vi "correlation tester.vi"() -> ()   [LabVIEW 2012]
uses:
  <vilib>/Utility/file.llb/Write To Spreadsheet File (DBL).vi
  <vilib>/vision/NI_Vision_Development_Module.lvlib
panel:
  in  "cc?":bool
  in  "report file name":path
  in  "error in":errorcluster
  out "error out":errorcluster
  out "Alignement peak":i32[](graph)
  out "Maximum quality per image":dbl[](graph)
  out "Alignment quality profile":sgl[](graph)
  in  "background image":path
  in  "Image sequence folder":path
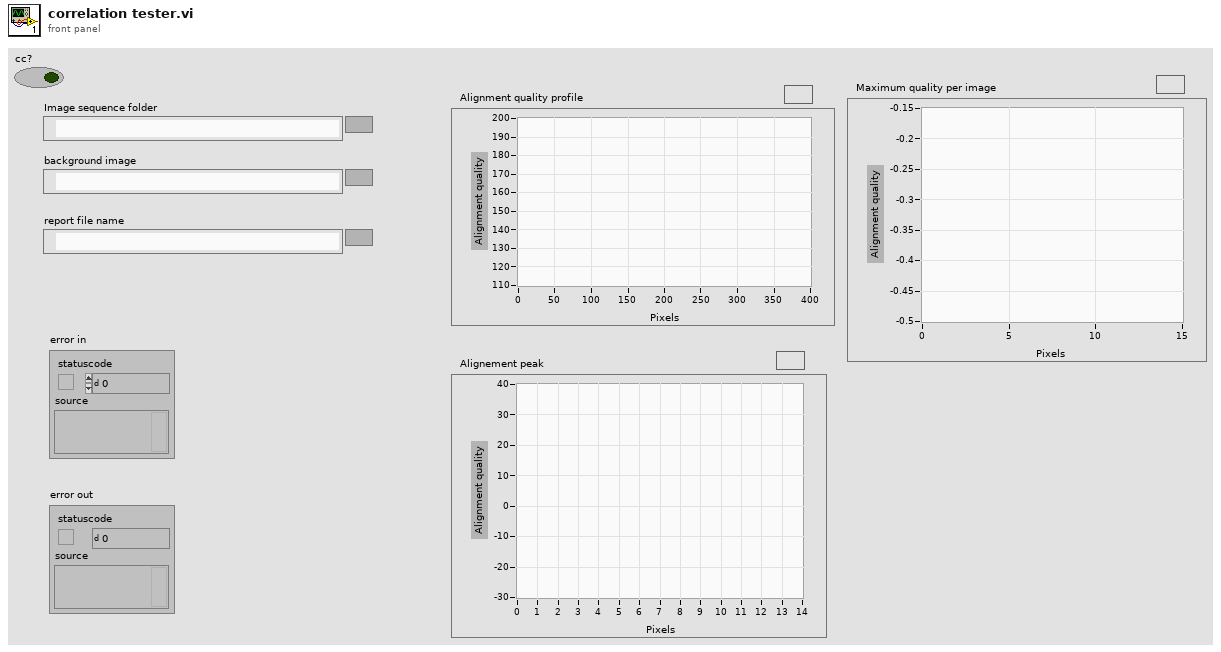
[diagram p1: front panel]
types:
  T1 = typedef "IMAQ Image.ctl" = refnum<image>
  T2 = typedef "ROI Descriptor" = cluster{"Global Rectangle":i32[], "Contours":cluster{"ID":enum32{"External", "Internal"}, "Type":u32, "Coordinates":i32[]}[]}
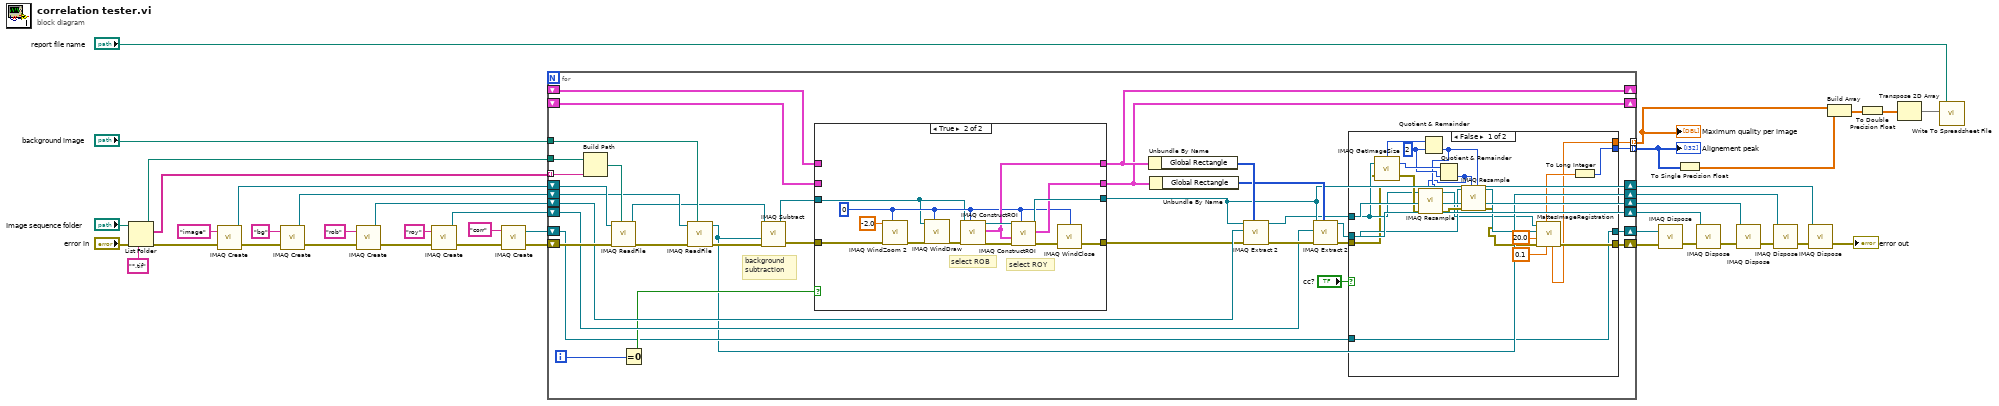
[diagram p0: block diagram]
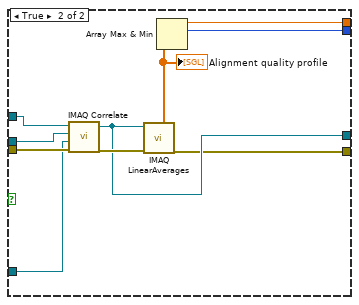
[diagram p2: hidden frame]
diagram:
  n1 = List Folder(path="Image sequence folder", pattern="*.tif", error in="error in") -> (path out=w22:path, filenames=w35:string[], error out=w40:errorcluster)  [unwired: 1 in, 1 out]
  n2 = call "IMAQ Create"("Image Name"="image", "error in (no error)"=w40) -> ("New Image"=w30:T1, "error out"=w39:errorcluster)  [unwired: 3 in]
  n3 = call "IMAQ Create"("Image Name"="bg", "error in (no error)"=w39) -> ("New Image"=w29:T1, "error out"=w38:errorcluster)  [unwired: 3 in]
  n4 = call "IMAQ Create"("Image Name"="rob", "error in (no error)"=w38) -> ("New Image"=w28:T1, "error out"=w37:errorcluster)  [unwired: 3 in]
  n5 = call "IMAQ Create"("Image Name"="roy", "error in (no error)"=w37) -> ("New Image"=w27:T1, "error out"=w26:errorcluster)  [unwired: 3 in]
  n6 = call "IMAQ Create"("Image Name"="corr", "error in (no error)"=w26) -> ("New Image"=w23:T1, "error out"=w25:errorcluster)  [unwired: 3 in]
  n7 = for {
    tunnel: w35 -> [w70] mode=indexing
    shift-right: [w43] -> w20
    shift-left: w25 -> [w75]
    shift-right: [w44] -> w14
    shift-left: w23 -> [w45]
    shift-right: [w48] -> w13
    shift-left: w27 -> [w63]
    shift-right: [w50] -> w12
    shift-left: w28 -> [w64]
    shift-right: [w41] -> w11
    shift-left: w29 -> [w68]
    shift-right: [w51] -> w10
    shift-left: w30 -> [w73]
    tunnel: w22 -> [w71]
    tunnel: "background image" -> [w72]
    shift-right: [w55] -> _
    shift-left: _ -> [w53]
    shift-right: [w54] -> _
    shift-left: _ -> [w52]
    tunnel: [w47] -> w7 mode=indexing
    tunnel: [w46] -> w8 mode=indexing
    i -> [w62]
    # "background\nsubtraction"
    n8 = Build Path(base path=w71, name or relative path=w70) -> (appended path=w69:path)
    n9 = call "IMAQ ReadFile"("File Path"=w69, "error in (no error)"=w75, "Image"=w73) -> ("error out"=w74:errorcluster, "Image Out"=w67:T1)  [unwired: 4 in, 3 out]
    n10 = Equal To 0?(x=w62) -> (x = 0?=w61:bool)
    n11 = call "IMAQ ReadFile"("File Path"=w72, "error in (no error)"=w74, "Image"=w68) -> ("error out"=w66:errorcluster, "Image Out"=w41:T1)  [unwired: 4 in, 3 out]
    n12 = call "IMAQ Subtract"("Image Src A"=w67, "Image Src B"=w41, "error in (no error)"=w66) -> ("Image Dst Out"=w58:T1, "error out"=w59:errorcluster)  [unwired: 4 in]
    n13 = case shown="True" w61 {
      tunnel: [w109 w115] -> w60
      tunnel: w59 -> [w109 w110]
      tunnel: [w108 w119] -> w51
      tunnel: w58 -> [w108 w111]
      tunnel: [w107 w118] -> w55
      tunnel: [w106 w117] -> w54
      tunnel: w53 -> [w107 _]
      tunnel: w52 -> [w106 _]
      frame False {
      }
      frame True {
        w112 = 0 ("Window Number (0...15)")
        # "select ROY"
        # "select ROB"
        n14 = call "IMAQ WindZoom 2"("Window Number (0...15)"=w112, "error in (no error)"=w110, "Zoom Factor"=sgl -2.0) -> ("error out"=w114:errorcluster)  [unwired: 5 in, 3 out]
        n15 = call "IMAQ WindDraw"("Window Number (0...15)"=w112, "Image"=w111) -> ()  [unwired: 8 in, 2 out]
        n16 = call "IMAQ ConstructROI"("Window Number (-1...15)"=w112, "error in (no error)"=w114, "Image"=w111) -> ("error out"=w120:errorcluster, "ROI Descriptor Out"=w118:T2, "Image Out (duplicate)"=w121:T1)  [unwired: 5 in, 1 out]
        n17 = call "IMAQ ConstructROI"("Window Number (-1...15)"=w112, "error in (no error)"=w120, "ROI Descriptor In (None)"=w118, "Image"=w121) -> ("error out"=w116:errorcluster, "ROI Descriptor Out"=w117:T2, "Image Out (duplicate)"=w119:T1)  [unwired: 4 in, 1 out]
        n18 = call "IMAQ WindClose"("Window Number (0...15)"=w112, "error in (no error)"=w116) -> ("error out"=w115:errorcluster)  [unwired: 4 in]
      }
    }
    n19 = Unbundle By Name(w55) -> ("Global Rectangle"=w57:i32[])
    n20 = Unbundle By Name(w54) -> ("Global Rectangle"=w56:i32[])
    n21 = call "IMAQ Extract 2"("Optional Rectangle"=w57, "error in (no error)"=w60, "Image Dst"=w64, "Image Src"=w51) -> ("error out"=w65:errorcluster, "Image Dst Out"=w50:T1)  [unwired: 6 in]
    n22 = call "IMAQ Extract 2"("Optional Rectangle"=w56, "error in (no error)"=w65, "Image Dst"=w63, "Image Src"=w51) -> ("error out"=w49:errorcluster, "Image Dst Out"=w48:T1)  [unwired: 6 in]
    n23 = case shown="False" "cc?" {
      tunnel: w50 -> [w84 w105]
      tunnel: w49 -> [w82 w104]
      tunnel: w48 -> [w86 w103]
      tunnel: [w92 w101] -> w47
      tunnel: [w93 w100] -> w46
      tunnel: w45 -> [w91 w98]
      tunnel: [w91 w97] -> w44
      tunnel: [w95 w96] -> w43
      frame False {
        w78 = 2 ("y")
        n24 = call "IMAQ GetImageSize"("Image"=w84, "error in (no error)"=w82) -> ("Y Resolution"=w80:i32, "X Resolution"=w79:i32, "error out"=w88:errorcluster)  [unwired: 2 in]
        n25 = Quotient & Remainder(x=w79, y=w78) -> (floor(x/y)=w77:i32)  [unwired: 1 out]
        n26 = Quotient & Remainder(x=w80, y=w78) -> (floor(x/y)=w76:i32)  [unwired: 1 out]
        n27 = call "IMAQ Resample"("X Resolution"=w77, "Y Resolution"=w76, "error in (no error)"=w88, "Image Src"=w84) -> ("error out"=w87:errorcluster, "Image Dst Out"=w83:T1)  [unwired: 6 in]
        n28 = call "IMAQ Resample"("X Resolution"=w77, "Y Resolution"=w76, "error in (no error)"=w87, "Image Src"=w86) -> ("error out"=w81:errorcluster, "Image Dst Out"=w85:T1)  [unwired: 6 in]
        n29 = call "MattesImageRegistration.vi"("Epsilon"=0.1, "error in (no error)"=w81, "Starting Radius"=20.0, "Moving image in"=w85, "Fixed image in"=w83) -> ("error out"=w95:errorcluster, "alignment quality"=w92:dbl, "x translation"=w94:dbl)  [unwired: 4 out]
        n30 = To Long Integer(number=w94) -> (32bit integer=w93:i32)
      }
      frame True {
        n31 = call "IMAQ Correlate"("Image Src"=w105, "Image Template"=w103, "Image Dst"=w98, "error in (no error)"=w104) -> ("Image Dst Out"=w97:T1, "error out"=w102:errorcluster)  [unwired: 3 in]
        n32 = call "IMAQ LinearAverages"("error in (no error)"=w102, "Image Src"=w97) -> ("error out"=w96:errorcluster, "X Axis Averages"=w99:sgl[])  [unwired: 5 in, 3 out]
        "Alignment quality profile" <- w99
        n33 = Array Max & Min(array=w99) -> (max value=w101:sgl, max index (indices)=w100:i32)  [unwired: 2 out]
      }
    }
  }
  "Maximum quality per image" <- w7
  "Alignement peak" <- w8
  n34 = call "IMAQ Dispose"("Image"=w14, "error in (no error)"=w20) -> ("error out"=w19:errorcluster)  [unwired: 4 in]
  n35 = To Single Precision Float(number=w8) -> (single precision float=w6:sgl[])
  n36 = call "IMAQ Dispose"("Image"=w13, "error in (no error)"=w19) -> ("error out"=w18:errorcluster)  [unwired: 4 in]
  n37 = call "IMAQ Dispose"("Image"=w12, "error in (no error)"=w18) -> ("error out"=w17:errorcluster)  [unwired: 4 in]
  n38 = call "IMAQ Dispose"("Image"=w11, "error in (no error)"=w17) -> ("error out"=w16:errorcluster)  [unwired: 4 in]
  n39 = call "IMAQ Dispose"("Image"=w10, "error in (no error)"=w16) -> ("error out"=→"error out":errorcluster)  [unwired: 4 in]
  n40 = Build Array(w7, w6) -> (w5:dbl[][])
  n41 = To Double Precision Float(number=w5) -> (double precision float=w4:dbl[][])
  n42 = Transpose 2D Array(2D array=w4) -> (transposed array=w1:dbl[][])
  n43 = call-poly <vilib>:"Write To Spreadsheet File.vi"("2D data"=w1, "file path (dialog if empty)"="report file name") -> ()  [unwired: 6 in, 1 out]
